vi "Write header (SubVI).vi"(8 "error in":errorcluster, 9 "Settings array in":i32[](array[numeric]), 10 "Append? Out":bool, 11 "Path in":path) -> (0 "error out":errorcluster, 3 "Path out":path)   [LabVIEW 2017, in "Fridge Software v2.1.lvlib"]
uses:
  Fridge Software v2.1.lvlib
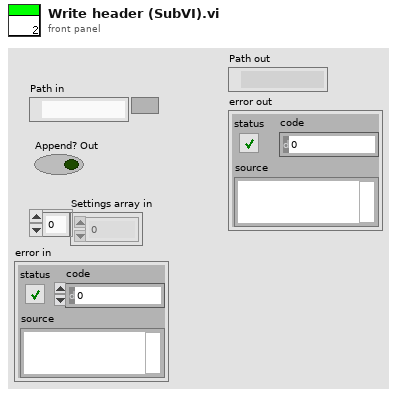
[diagram p1: front panel]
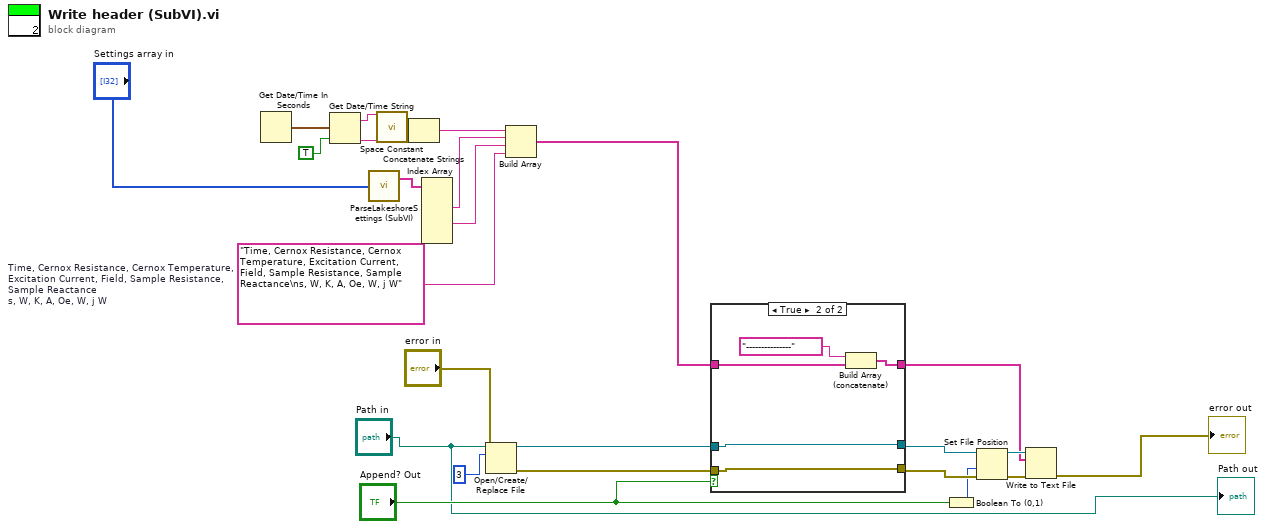
[diagram p0: block diagram]
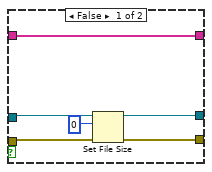
[diagram p2: hidden frame]
diagram:
  w4 = "Time, Cernox Resistance, Cernox Temperature, Excitation Current, Field, Sample Resistance, Sample Reactance\ns, W, K, A, Oe, W, j W"  # Time, Cernox Resistance, Cernox Temperature, Excitation Current, Field, Sample Resistance, Sample Reactance s, W, K, A, Oe, W, j W
  n1 = Get Date/Time In Seconds() -> (seconds since 1Jan1904=w20:timestamp)
  n2 = Get Date/Time String(seconds (now)=w20, want seconds? (F)=TRUE) -> (date string=w11:string, time string=w7:string)  [unwired: 1 in]
  n3 = call "ParseLakeshoreSettings (SubVI).vi"("Settings array in"="Settings array in") -> ("Array"=w19:string[])  [unwired: 1 out]
  n4 = call <vilib>:"Space Constant.vi"() -> ("String"=w6:string)
  n5 = Concatenate Strings(w11, w6, w7) -> (w10:string)
  n6 = Index Array(array=w19) -> (element #2=w9:string, element #4=w8:string)  [unwired: 6 in, 4 out]
  n7 = Open/Create/Replace File(file path (use dialog)="Path in", error in="error in", operation (0:open)=3) -> (refnum out=w22:refnum<file>, error out=w23:errorcluster)  [unwired: 3 in, 1 out]
  n8 = Build Array(w10, w9, w8, w4) -> (w13:string[])
  n9 = case shown="True" "Append? Out" {
    tunnel: w22 -> [w31 w36]
    tunnel: w23 -> [w29 w35]
    tunnel: [w28 w35] -> w24
    tunnel: [w27 w36] -> w25
    tunnel: w13 -> [w26 w34]
    tunnel: [w26 w32] -> w12
    frame False {
      n10 = Set File Size(4:w29, 6:0, 7:w31) -> (0:w28:errorcluster, 3:w27:refnum<file>)
    }
    frame True {
      n11 = Build Array (concatenate)("---------------", w34) -> (w32:string[])
    }
  }
  n12 = Boolean To (0,1)(Boolean="Append? Out") -> (0, 1=w14:i16)
  n13 = Set File Position(refnum=w25, from (0:start)=w14, error in=w24) -> (refnum out=w18:refnum<file>, error out=w16:errorcluster)  [unwired: 1 in]
  n14 = Write to Text File(file (use dialog)=w18, text=w12, error in=w16) -> (error out=→"error out":errorcluster)  [unwired: 1 in, 2 out]
  "Path out" <- "Path in"
